vi "Write Greater_.vi"(8 "error in (no error)":errorcluster, 10 "Greater?":bool, 11 "AssertCompareValue in":refnum<class "AssertCompareValue.lvclass">) -> (0 "error out":errorcluster, 3 "AssertCompareValue out":refnum<class "AssertCompareValue.lvclass">)   [LabVIEW 2021, in "Bananas.lvlib" / "AssertCompareValue.lvclass"]
uses:
  AssertCompareValue.lvclass
  AssertCompareValue.lvclass/AssertCompareValue.ctl
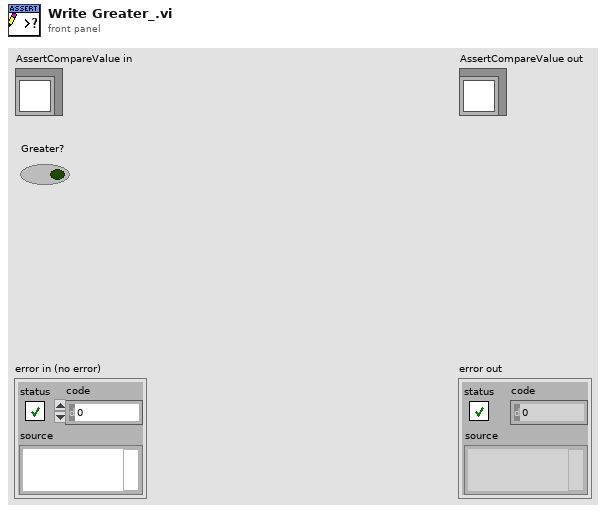
[diagram p1: front panel]
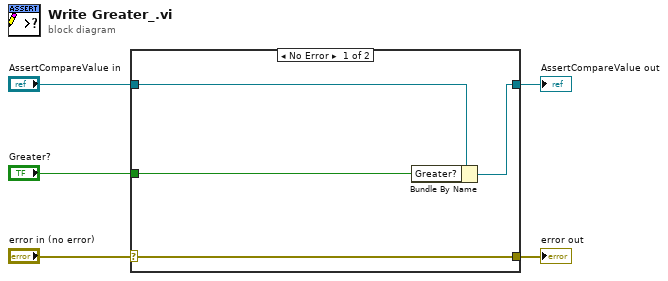
[diagram p0: block diagram]
diagram:
  n1 = case shown="No Error" "error in (no error)" {
    selector: "error in (no error)" -> [w9 w10]
    tunnel: [w9 w10] -> w4
    tunnel: [w7 w11] -> w2
    tunnel: "AssertCompareValue in" -> [w8 w11]
    tunnel: "Greater?" -> [w6 _]
    frame No Error {
      n2 = Bundle By Name(cluster=w8, "Greater?"=w6) -> (w7:refnum<class "AssertCompareValue.lvclass">)
    }
    frame Error {
    }
  }
  "error out" <- w4
  "AssertCompareValue out" <- w2
